vi "Save CAN data.vi"(4 "Frames":refnum<vi>, 5 "DBC path":refnum<vi>, 6 "Tree Data":refnum<vi>, 7 "Headers":string[](array[string]), 8 "error in":errorcluster, 9 "Bus Type":refnum<vi>, 10 "Format":refnum<vi>, 11 "Path":refnum<vi>) -> (0 "error out":errorcluster, 3 "Status":string)   [LabVIEW 2025, in "CAN-LIN Raw Bus Capture UI.lvlib"]
doc: "Save the data from the trace table to the path folder in a pre-defined file name format, and with the defined file format."
uses:
  CAN-LIN Raw Bus Capture UI.lvlib
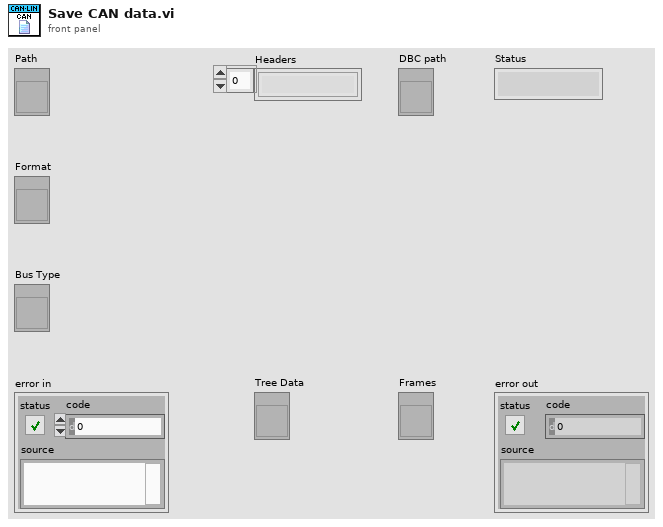
[diagram p1: front panel]
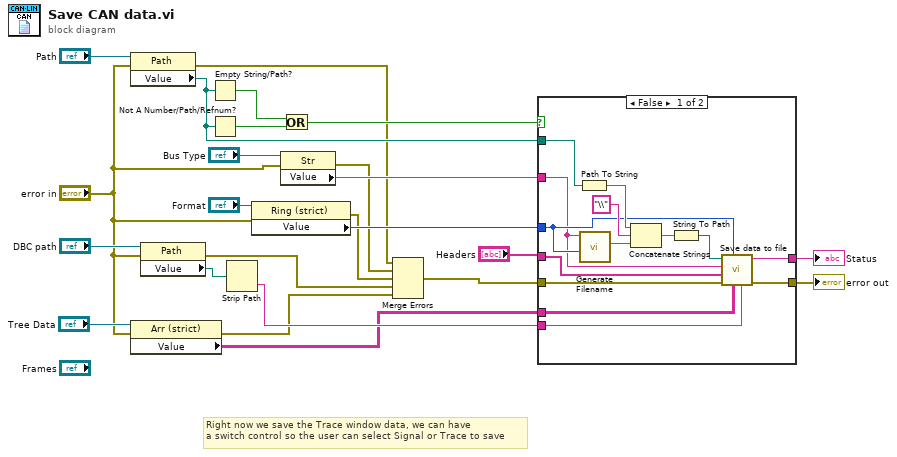
[diagram p0: block diagram]
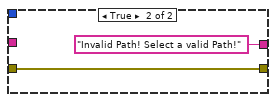
[diagram p2: hidden frame]
diagram:
  # "Right now we save the Trace window data, we can have\na switch control so the user can select Signal or Trace to save"
  n1 = property class="Path"(reference="Path", error in="error in") -> (error out=w8:errorcluster, "Value"=w16:path)  [unwired: 1 out]
  n2 = property class="Arr (strict)"(reference="Tree Data", error in="error in") -> (error out=w2:errorcluster, "Value"=w1:string[][])  [unwired: 1 out]
  n3 = property class="Path"(reference="DBC path", error in="error in") -> (error out=w5:errorcluster, "Value"=w10:path)  [unwired: 1 out]
  n4 = Empty String/Path?(string/path=w16) -> (empty?=w22:bool)
  n5 = Not A Number/Path/Refnum?(number/path/refnum=w16) -> (NaN/Path/Refnum?=w23:bool)
  n6 = Strip Path(path=w10) -> (name=w9:string)  [unwired: 1 out]
  n7 = property class="Ring (strict)"(reference="Format", error in="error in") -> (error out=w6:errorcluster, "Value"=w15:u16)  [unwired: 1 out]
  n8 = property class="Str"(reference="Bus Type", error in="error in") -> (error out=w7:errorcluster, "Value"=w14:string)  [unwired: 1 out]
  n9 = Or(x=w22, y=w23) -> (x .or. y?=w24:bool)
  n10 = Merge Errors(w8, w7, w6, w5, w2) -> (w12:errorcluster)
  n11 = case shown="False" w24 {
    tunnel: w16 -> [w35 _]
    tunnel: "Headers" -> [w38 _]
    tunnel: w12 -> [w37 w40]
    tunnel: [w36 w40] -> w21
    tunnel: w15 -> [w29 _]
    tunnel: [w28 "Invalid Path! Select a valid Path!" ("message")] -> w19
    tunnel: w14 -> [w27 _]
    tunnel: w9 -> [w26 _]
    tunnel: w1 -> [w25 _]
    frame False {
      n12 = Path To String(path=w35) -> (string=w34:string)
      n13 = call "Generate Filename.vi"("format  in"=w29, "bustype in"=w27) -> ("filename"=w33:string)  [unwired: 9 in]
      n14 = Concatenate Strings(w34, "\\", w33) -> (w31:string)
      n15 = String To Path(string=w31) -> (path=w30:path)
      n16 = call "Save data to file.vi"("DBC file name"=w26, "Captured Data"=w25, "SAVE FORMAT"=w29, "error in"=w37, "Headers"=w38, "Bus Type"=w27, "Path"=w30) -> ("error out"=w36:errorcluster, "message"=w28:string)  [unwired: 3 in]
    }
    frame True {
    }
  }
  "error out" <- w21
  "Status" <- w19
